vi "Switch Interface.vi"() -> ()   [LabVIEW 2011]
uses:
  SubVI/Pumps_Valves_Dependencies_Global.vi
panel:
  in  "Mode of Operation":bool
  out "Towing tank Volume":dbl
  out "Salt Saturator":dbl(slide) scale=0.0..100.0
  out "B":dbl(slide) scale=0.0..100.0
  out "A":dbl(slide) scale=0.0..100.0
  out "Density Meter":dbl
  out "D":dbl(slide) scale=0.0..100.0
  out "C":dbl(slide) scale=0.0..100.0
  in  "?":bool
  in  "Valve Power":bool
  in  "Pump Power":bool
  in  "Main Rack Power":bool
  in  "V34":bool
  in  "V32":bool
  in  "V19":bool
  in  "V33":bool
  in  "V18":bool
  in  "V20":bool
  in  "V26":bool
  in  "V25":bool
  in  "V24":bool
  in  "V23":bool
  in  "V22":bool
  in  "V21":bool
  in  "V27":bool
  in  "V28":bool
  in  "V31":bool
  in  "V13":bool
  in  "V15":bool
  in  "V11":bool
  in  "V10":bool
  in  "V9":bool
  in  "V14":bool
  in  "V8":bool
  in  "V6":bool
  in  "V7":bool
  in  "V12":bool
  in  "V5":bool
  in  "V4":bool
  in  "V30":bool
  in  "V29":bool
  in  "Pump D":bool
  in  "Pump C":bool
  in  "Pump B":bool
  in  "Pump A":bool
  out "Fresh Water":dbl(slide) scale=0.0..10.0
  out "Brine":dbl(slide) scale=0.0..10.0
  # "DRAIN"
  # "DRAIN"
  # "WATER SUPPLY"
  # "DRAIN"
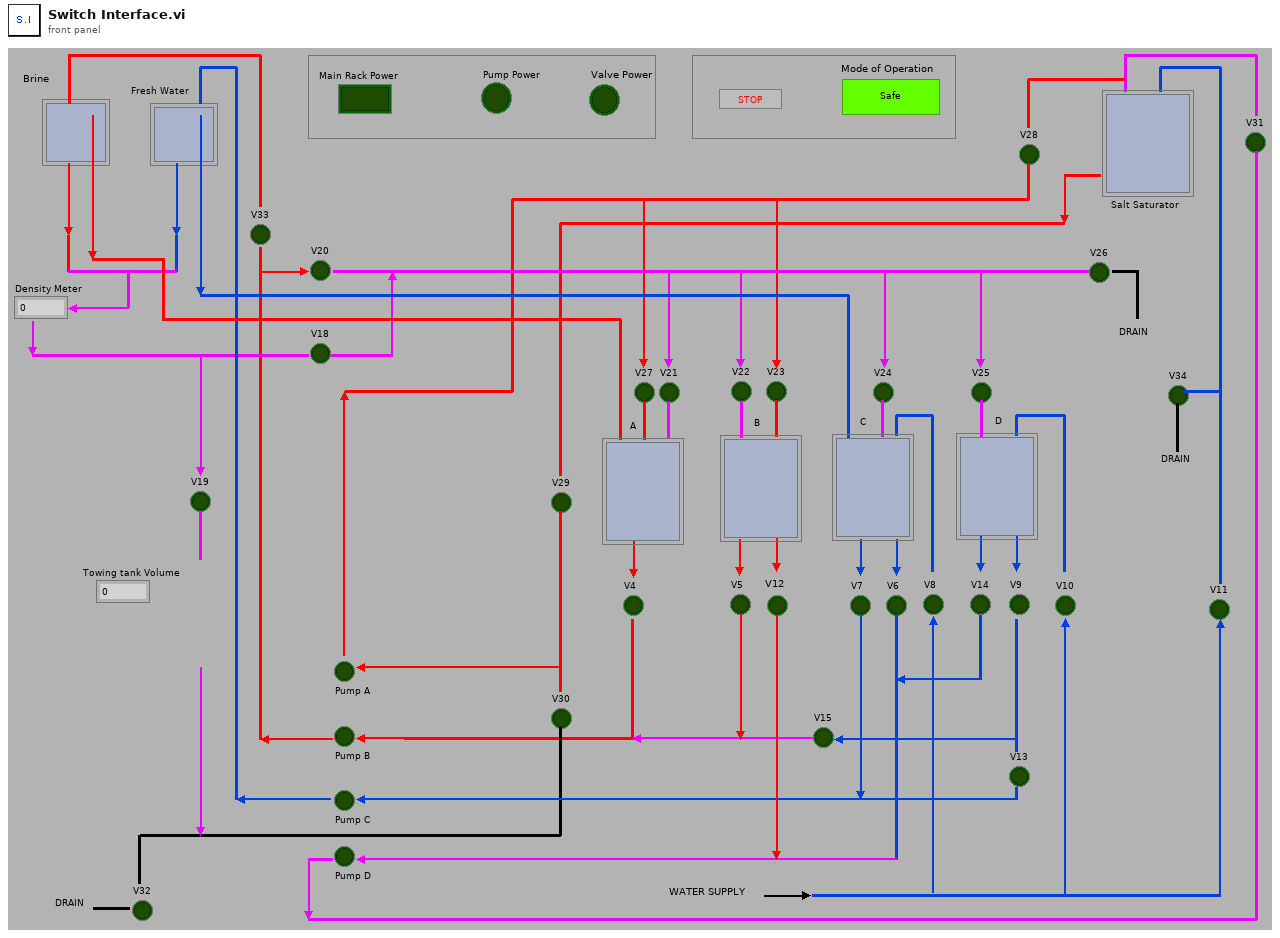
[diagram p1: front panel]
types:
  T1 = typedef "Valve_Pump.ctl" = enum16{"Main Rack Power", "Pump Power", "Valve Power", "V4", "V5", "V6", "V7", "V8", "V9", "V10", "V11", "V12", "V13", "V14", "V15", "V18", "V19", "V20", "V21", "V22", "V23", "V24", "V25", "V26", "V27", "V28", "V29", "V30", "V31", "V32", "V33", "V34", "Pump A", "Pump B", "Pump C", "Pump D"}
  T2 = cluster{"Height Array[0]":dbl, "Height Array[1]":dbl, "Height Array[2]":dbl, "Height Array[3]":dbl, "Height Array[4]":dbl}
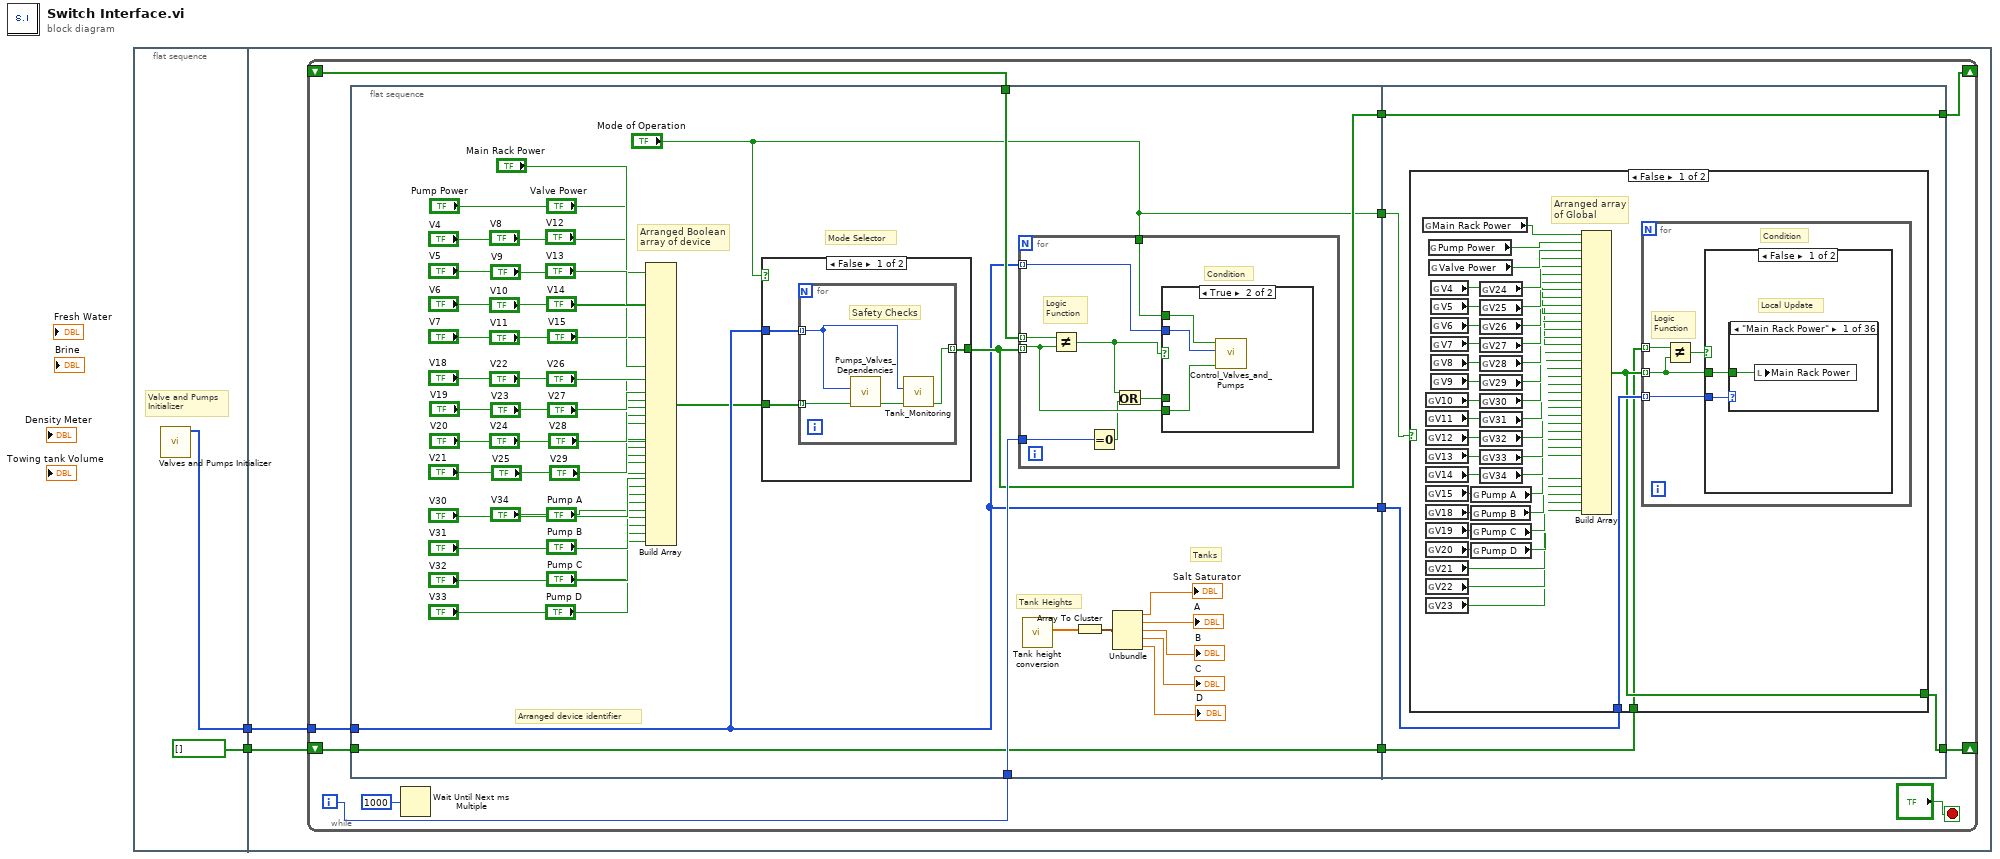
[diagram p0: block diagram]
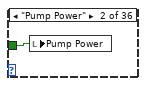
[diagram p4: hidden frame]
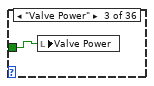
[diagram p5: hidden frame]
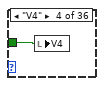
[diagram p6: hidden frame]
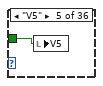
[diagram p7: hidden frame]
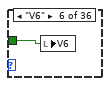
[diagram p8: hidden frame]
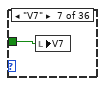
[diagram p9: hidden frame]
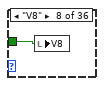
[diagram p10: hidden frame]
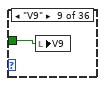
[diagram p11: hidden frame]
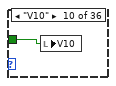
[diagram p12: hidden frame]
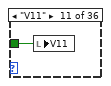
[diagram p13: hidden frame]
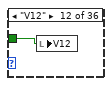
[diagram p14: hidden frame]
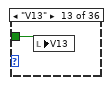
[diagram p15: hidden frame]
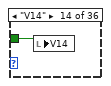
[diagram p16: hidden frame]
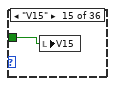
[diagram p17: hidden frame]
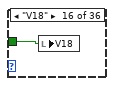
[diagram p18: hidden frame]
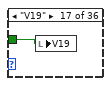
[diagram p19: hidden frame]
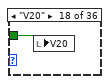
[diagram p20: hidden frame]
diagram:
  n1 = flat-sequence {
    tunnel: [w3] -> w2
    tunnel: [bool[] []] -> w1
    tunnel: w2 -> [w6]
    tunnel: w1 -> [w5]
    frame #0 {
      # "Valve and Pumps\nInitializer"
      n2 = call "Valves and Pumps Initializer.vi"() -> ("Devices"=w3:T1[])  [unwired: 11 in]
    }
    frame #1 {
      n3 = while {
        shift-right: [w11] -> _
        shift-left: _ -> [w17]
        tunnel: w6 -> [w10]
        shift-right: [w9] -> _
        shift-left: w5 -> [w7]
        i -> [w16]
        stop <- "?" stop-if-true
        n4 = flat-sequence {
          tunnel: w17 -> [w68]
          tunnel: w16 -> [w67]
          tunnel: [w51] -> w14
          tunnel: [w50] -> w13
          tunnel: ["Mode of Operation"] -> w12
          tunnel: w10 -> [w50]
          tunnel: [w49] -> w8
          tunnel: w7 -> [w49]
          tunnel: [w92] -> w11
          tunnel: w14 -> [w92]
          tunnel: w13 -> [w91]
          tunnel: w12 -> [w90]
          tunnel: [w89] -> w9
          tunnel: w8 -> [w88]
          frame #0 {
            # "Tanks"
            # "Arranged device identifier"
            # "Tank Heights"
            # "Arranged Boolean \narray of device"
            # "Mode Selector"
            n5 = Build Array("Main Rack Power", "Pump Power", "Valve Power", "V4", "V5", "V6", "V7", "V8", "V9", "V10", "V11", "V12", "V13", "V14", "V15", "V18", "V19", "V20", "V21", "V22", "V23", "V24", "V25", "V26", "V27", "V28", "V29", "V30", "V31", "V32", "V33", "V34", "Pump A", "Pump B", "Pump C", "Pump D") -> (w19:bool[])
            n6 = case shown="False" "Mode of Operation" {
              tunnel: w19 -> [w71 w76]
              tunnel: [w70 w76] -> w51
              tunnel: w50 -> [w69 _]
              frame False {
                n7 = for {
                  tunnel: w71 -> [w75] mode=indexing
                  tunnel: [w72] -> w70 mode=indexing
                  tunnel: w69 -> [w74] mode=indexing
                  # "Safety Checks"
                  n8 = call "Pumps_Valves_Dependencies.vi"("Set state:"=w75, "Device"=w74) -> ("State"=w73:bool)  [unwired: 9 in]
                  n9 = call "Tank_Monitoring.vi"("Set state:"=w73, "Device"=w74) -> ("Set"=w72:bool)  [unwired: 9 in]
                }
              }
              frame True {
              }
            }
            n10 = for {
              tunnel: w50 -> [w82] mode=indexing
              tunnel: w51 -> [w81] mode=indexing
              tunnel: w68 -> [w80] mode=indexing
              tunnel: w67 -> [w78]
              tunnel: "Mode of Operation" -> [w77]
              # "Logic\nFunction"
              # "Condition"
              n11 = Not Equal?(x=w80, y=w81) -> (x != y?=w84:bool)
              n12 = Equal To 0?(x=w78) -> (x = 0?=w79:bool)
              n13 = Or(x=w84, y=w79) -> (x .or. y?=w83:bool)
              n14 = case shown="True" w84 {
                tunnel: w82 -> [_ w87]
                tunnel: w83 -> [_ _]
                tunnel: w81 -> [_ w86]
                tunnel: w77 -> [_ w85]
                frame False {
                }
                frame True {
                  n15 = call "Control_Valves_and_Pumps.vi"("Set state:"=w86, "Device"=w87, "Mode of Operation"=w85) -> ()  [unwired: 9 in]
                }
              }
            }
            n16 = call "Tank height conversion.vi"() -> ("Height Array"=w42:dbl[])  [unwired: 11 in]
            n17 = Array To Cluster(array=w42) -> (cluster=w48:T2)
            n18 = Unbundle(w48) -> ("Height Array[0]"=→"Salt Saturator":dbl, "Height Array[1]"=→"A":dbl, "Height Array[2]"=→"B":dbl, "Height Array[3]"=→"C":dbl, "Height Array[4]"=→"D":dbl)
          }
          frame #1 {
            n19 = case shown="False" w90 {
              tunnel: w91 -> [w131 _]
              tunnel: [w94 w174] -> w89
              tunnel: w88 -> [w93 w174]
              frame False {
                # "Arranged array\nof Global"
                n20 = global read "Pumps_Valves_Dependencies_Global.vi" "Main Rack Power"() -> (w130:bool)
                n21 = global read "Pumps_Valves_Dependencies_Global.vi" "V10"() -> (w121:bool)
                n22 = global read "Pumps_Valves_Dependencies_Global.vi" "V11"() -> (w120:bool)
                n23 = global read "Pumps_Valves_Dependencies_Global.vi" "V12"() -> (w119:bool)
                n24 = global read "Pumps_Valves_Dependencies_Global.vi" "V13"() -> (w118:bool)
                n25 = global read "Pumps_Valves_Dependencies_Global.vi" "V14"() -> (w117:bool)
                n26 = global read "Pumps_Valves_Dependencies_Global.vi" "V15"() -> (w116:bool)
                n27 = global read "Pumps_Valves_Dependencies_Global.vi" "V18"() -> (w115:bool)
                n28 = global read "Pumps_Valves_Dependencies_Global.vi" "V19"() -> (w114:bool)
                n29 = global read "Pumps_Valves_Dependencies_Global.vi" "V20"() -> (w113:bool)
                n30 = global read "Pumps_Valves_Dependencies_Global.vi" "V21"() -> (w112:bool)
                n31 = global read "Pumps_Valves_Dependencies_Global.vi" "V22"() -> (w111:bool)
                n32 = global read "Pumps_Valves_Dependencies_Global.vi" "V23"() -> (w110:bool)
                n33 = global read "Pumps_Valves_Dependencies_Global.vi" "Pump Power"() -> (w129:bool)
                n34 = global read "Pumps_Valves_Dependencies_Global.vi" "Valve Power"() -> (w128:bool)
                n35 = global read "Pumps_Valves_Dependencies_Global.vi" "V4"() -> (w127:bool)
                n36 = global read "Pumps_Valves_Dependencies_Global.vi" "V5"() -> (w126:bool)
                n37 = global read "Pumps_Valves_Dependencies_Global.vi" "V6"() -> (w125:bool)
                n38 = global read "Pumps_Valves_Dependencies_Global.vi" "V7"() -> (w124:bool)
                n39 = global read "Pumps_Valves_Dependencies_Global.vi" "V8"() -> (w123:bool)
                n40 = global read "Pumps_Valves_Dependencies_Global.vi" "V9"() -> (w122:bool)
                n41 = global read "Pumps_Valves_Dependencies_Global.vi" "Pump A"() -> (w98:bool)
                n42 = global read "Pumps_Valves_Dependencies_Global.vi" "Pump B"() -> (w97:bool)
                n43 = global read "Pumps_Valves_Dependencies_Global.vi" "Pump C"() -> (w96:bool)
                n44 = global read "Pumps_Valves_Dependencies_Global.vi" "Pump D"() -> (w95:bool)
                n45 = global read "Pumps_Valves_Dependencies_Global.vi" "V24"() -> (w109:bool)
                n46 = global read "Pumps_Valves_Dependencies_Global.vi" "V25"() -> (w108:bool)
                n47 = global read "Pumps_Valves_Dependencies_Global.vi" "V26"() -> (w107:bool)
                n48 = global read "Pumps_Valves_Dependencies_Global.vi" "V27"() -> (w106:bool)
                n49 = global read "Pumps_Valves_Dependencies_Global.vi" "V28"() -> (w105:bool)
                n50 = global read "Pumps_Valves_Dependencies_Global.vi" "V29"() -> (w104:bool)
                n51 = global read "Pumps_Valves_Dependencies_Global.vi" "V30"() -> (w103:bool)
                n52 = global read "Pumps_Valves_Dependencies_Global.vi" "V31"() -> (w102:bool)
                n53 = global read "Pumps_Valves_Dependencies_Global.vi" "V32"() -> (w101:bool)
                n54 = global read "Pumps_Valves_Dependencies_Global.vi" "V33"() -> (w100:bool)
                n55 = global read "Pumps_Valves_Dependencies_Global.vi" "V34"() -> (w99:bool)
                n56 = Build Array(w130, w129, w128, w127, w126, w125, w124, w123, w122, w121, w120, w119, w118, w117, w116, w115, w114, w113, w112, w111, w110, w109, w108, w107, w106, w105, w104, w103, w102, w101, w100, w99, w98, w97, w96, w95) -> (w94:bool[])
                n57 = for {
                  tunnel: w94 -> [w133] mode=indexing
                  tunnel: w131 -> [w134] mode=indexing
                  tunnel: w93 -> [w132] mode=indexing
                  # "Logic\nFunction"
                  # "Condition"
                  n58 = Not Equal?(x=w132, y=w133) -> (x != y?=w135:bool)
                  n59 = case shown="False" w135 {
                    tunnel: w134 -> [w137 _]
                    tunnel: w133 -> [w136 _]
                    frame False {
                      # "Local Update"
                      n60 = case shown="\"Main Rack Power\"" w137 {
                        tunnel: w136 -> [w138 w139 w140 w141 w142 w143 w144 w145 w146 w147 w148 w149 w150 w151 w152 w153 w154 w155 w156 w157 w158 w159 w160 w161 w162 w163 w164 w165 w166 w167 w168 w169 w170 w171 w172 w173]
                        frame "Main Rack Power" {
                          n61 = local write "Main Rack Power"(w138) -> ()
                        }
                        frame "Pump Power" {
                          n62 = local write "Pump Power"(w139) -> ()
                        }
                        frame "Valve Power" {
                          n63 = local write "Valve Power"(w140) -> ()
                        }
                        frame "V4" {
                          n64 = local write "V4"(w141) -> ()
                        }
                        frame "V5" {
                          n65 = local write "V5"(w142) -> ()
                        }
                        frame "V6" {
                          n66 = local write "V6"(w143) -> ()
                        }
                        frame "V7" {
                          n67 = local write "V7"(w144) -> ()
                        }
                        frame "V8" {
                          n68 = local write "V8"(w145) -> ()
                        }
                        frame "V9" {
                          n69 = local write "V9"(w146) -> ()
                        }
                        frame "V10" {
                          n70 = local write "V10"(w147) -> ()
                        }
                        frame "V11" {
                          n71 = local write "V11"(w148) -> ()
                        }
                        frame "V12" {
                          n72 = local write "V12"(w149) -> ()
                        }
                        frame "V13" {
                          n73 = local write "V13"(w150) -> ()
                        }
                        frame "V14" {
                          n74 = local write "V14"(w151) -> ()
                        }
                        frame "V15" {
                          n75 = local write "V15"(w152) -> ()
                        }
                        frame "V18" {
                          n76 = local write "V18"(w153) -> ()
                        }
                        frame "V19" {
                          n77 = local write "V19"(w154) -> ()
                        }
                        frame "V20" {
                          n78 = local write "V20"(w155) -> ()
                        }
                        frame "V21" {
                          n79 = local write "V21"(w156) -> ()
                        }
                        frame "V22" {
                          n80 = local write "V22"(w157) -> ()
                        }
                        frame "V23" {
                          n81 = local write "V23"(w158) -> ()
                        }
                        frame "V24" {
                          n82 = local write "V24"(w159) -> ()
                        }
                        frame "V25" {
                          n83 = local write "V25"(w160) -> ()
                        }
                        frame "V26" {
                          n84 = local write "V26"(w161) -> ()
                        }
                        frame "V27" {
                          n85 = local write "V27"(w162) -> ()
                        }
                        frame "V28" {
                          n86 = local write "V28"(w163) -> ()
                        }
                        frame "V29" {
                          n87 = local write "V29"(w164) -> ()
                        }
                        frame "V30" {
                          n88 = local write "V30"(w165) -> ()
                        }
                        frame "V31" {
                          n89 = local write "V31"(w166) -> ()
                        }
                        frame "V32" {
                          n90 = local write "V32"(w167) -> ()
                        }
                        frame "V33" {
                          n91 = local write "V33"(w168) -> ()
                        }
                        frame "V34" {
                          n92 = local write "V34"(w169) -> ()
                        }
                        frame "Pump A" {
                          n93 = local write "Pump A"(w170) -> ()
                        }
                        frame "Pump B" {
                          n94 = local write "Pump B"(w171) -> ()
                        }
                        frame "Pump C" {
                          n95 = local write "Pump C"(w172) -> ()
                        }
                        frame "Pump D" {
                          n96 = local write "Pump D"(w173) -> ()
                        }
                      }
                    }
                    frame True {
                    }
                  }
                }
              }
              frame True {
              }
            }
          }
        }
        n97 = Wait Until Next ms Multiple(millisecond multiple=u32 1000) -> ()  [unwired: 1 out]
      }
    }
  }
